vi "serialization tests.vi"() -> ()   [LabVIEW 2013, in "Tag Bus Web Interface tests.lvlib"]
uses:
  Tag Bus Web Interface tests.lvlib
  <vilib>/NI/Tag Bus Module Framework/channel/channel classification.ctl
  <vilib>/NI/Tag Bus Module Framework/channel/TBM channel.lvclass
  configuration/Tag Bus Web Interface configuration.lvclass
  <vilib>/NI/Configuration Framework/serializable configuration/NISE_CEF_serializable configuration.lvclass
panel:
  out "channels equal":bool
  out "no error":errorcluster
  out "no error":errorcluster
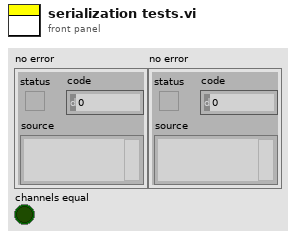
[diagram p1: front panel]
types:
  T1 = typedef "TBM channel.lvclass/channel classification.ctl" = enum16{"input data", "output data", "processing parameter", "processing result"}
  T2 = typedef "tag bus.lvlib/tag descriptor.lvclass/Data Type.ctl" = enum16{"Double", "Single", "I64", "I32", "I16", "I8", "U64", "U32", "U16", "U8", "Boolean", "String", "Array of Double", "Array of Single", "Array of I64", "Array of I32", "Array of I16", "Array of I8", "Array of U64", "Array of U32", "Array of U16", "Array of U8", "Array of Boolean", "Array of String"}
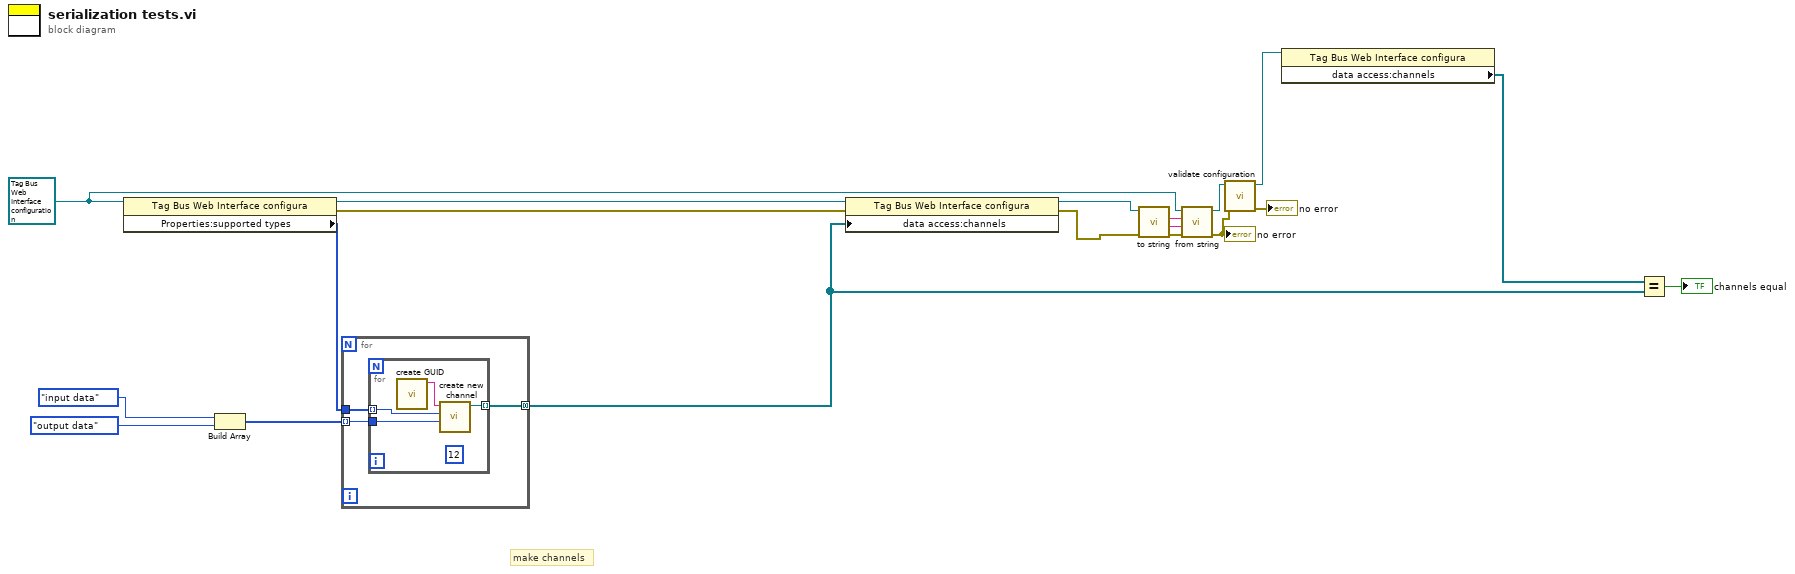
[diagram p0: block diagram]
diagram:
  w5 = refnum<class "Tag Bus Web Interface configuration.lvclass"> refnum ("tag bus configurable plugin module configuration")
  # "make channels"
  n1 = property class="Tag Bus Web Interface configura"(reference=w5) -> (reference out=w8:refnum<class "Tag Bus Web Interface configuration.lvclass">, error out=w1:errorcluster, "Properties:supported types"=w11:T2[])  [unwired: 1 in]
  n2 = Build Array(channel_classification."input data" ("channel classification"), channel_classification."output data" ("channel classification")) -> (w12:T1[])
  n3 = for {
    tunnel: w12 -> [w22] mode=indexing
    tunnel: [w21] -> w3 mode=concatenating
    tunnel: w11 -> [w20]
    n4 = for {
      tunnel: w22 -> [w25]
      tunnel: [w26] -> w21 mode=indexing
      tunnel: w20 -> [w24] mode=indexing
      (unwired) 12
      n5 = call <vilib>:"create GUID.vi"() -> ("uuid"=w23:string)  [unwired: 11 in]
      n6 = call <vilib>:"create new channel.vi"("channel classification"=w25, "data type"=w24, "channel name"=w23) -> ("channel"=w26:refnum<class "TBM channel.lvclass">)  [unwired: 8 in]
    }
  }
  n7 = property class="Tag Bus Web Interface configura"(reference=w8, error in=w1, "data access:channels"=w3) -> (reference out=w4:refnum<class "Tag Bus Web Interface configuration.lvclass">, error out=w2:errorcluster)
  n8 = call-dynamic "to string.vi"("error in"=w2, "Tag Bus Web Interface configuration in"=w4) -> ("error out"=w19:errorcluster, "data"=w18:string, "version"=w17:string)  [unwired: 6 in, 1 out]
  n9 = call-dynamic "from string.vi"("error in"=w19, "data"=w18, "version"=w17, "Tag Bus Web Interface configuration in"=w5) -> ("error out"=w10:errorcluster, "Tag Bus Web Interface configuration out"=w16:refnum<class "Tag Bus Web Interface configuration.lvclass">)  [unwired: 6 in]
  "no error" <- w10
  n10 = call-dynamic "validate configuration.vi"("error in"=w10, "Tag Bus Web Interface configuration in"=w16) -> ("error out"=→"no error":errorcluster, "Tag Bus Web Interface configuration out"=w7:refnum<class "Tag Bus Web Interface configuration.lvclass">)  [unwired: 8 in]
  n11 = property class="Tag Bus Web Interface configura"(reference=w7) -> ("data access:channels"=w6:refnum<class "TBM channel.lvclass">[])  [unwired: 1 in, 2 out]
  n12 = Equal?(x=w6, y=w3) -> (x = y?=→"channels equal":bool)
